vi "Measure.vi"(0 "eye scan single point":refnum<class "niHighSpeedSerial Eye Scan Single Point v1 Host.lvclass">, 5 "timeout (100 ms)":dbl=0.1, 11 "error in":errorcluster) -> (4 "eye scan single point out":refnum<class "niHighSpeedSerial Eye Scan Single Point v1 Host.lvclass">, 6 "bit error ratio":dbl, 8 "sample count":u64, 10 "error count":u64, 13 "timed out?":bool, 14 "done?":bool, 15 "error out":errorcluster)   [LabVIEW 2014, in "niHighSpeedSerial Eye Scan Single Point v1 Host.lvclass"]
doc: "Returns the Bit Error Rate, sample count, and error count on the point previously specified.\nThis VI returns under the following conditions, whichever comes first:\n1) The Eye Scan engine has completed measuring the point.\n2) The <b>timeout</b> is reached.\n\n<B>Input Parameters</B>\n\n<B>eye scan single point</B> takes in a reference to your session from the previous VI.\n\n<B>timeout (100 ms)</B> The amount of time (in seconds) before timing timing out.\nSpecifying '-1' prevents 'timed out' from ever returning true.\n\n<B>error in</B> describes error conditions that occur before this node runs. This input provides standard 'error in' functionality.\n\n<B>Output Parameters</B>\n\n<B>eye scan single point out</B> passes a reference to your session to the next VI.\n\n<B>bit error rate</B> is the calculated statistical bit error rate based on the number of error counts and sample counts received.\n\n<B>sample count</B> is the number of samples that have been measured on this point.\n\n<B>error count</B> is the number of errors that have been measured on this point.\n\n<B>timed out?</B> returns true if at least 'timeout' amount of time has passed.\n\n<B>done?</B> returns true if the Eye Scan algorithm has completed measuring all points.\n\n<B>error out</B> contains error information. This output provides standard 'error out' functionality."
uses:
  <instrlib>/niHighSpeedSerial/Eye Scan/v1/Host/Impl/Single Point/niHighSpeedSerial Eye Scan Single Point v1 Host.lvclass
  <instrlib>/niHighSpeedSerial/Eye Scan/v1/Host/Impl/Single Point/niHighSpeedSerial Eye Scan Single Point v1 Host.lvclass/niHighSpeedSerial Eye Scan Single Point v1 Host.ctl
  <vilib>/Utility/error.llb/Error Cluster From Error Code.vi
  <vilib>/ErrorRing/Error Ring.xnode
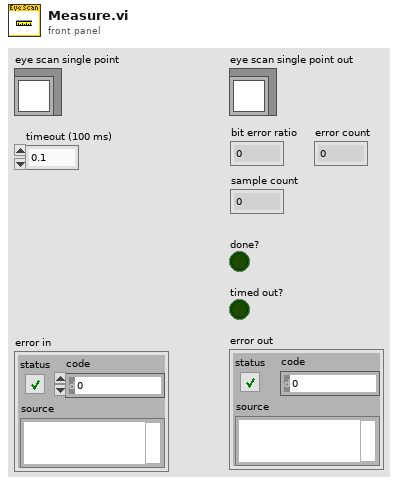
[diagram p1: front panel]
types:
  T1 = typedef "niHighSpeedSerial Eye Scan Single Point v1 Host.lvclass/Private Data.ctl" = cluster{"GTX2_CHANNEL register map":refnum<class "GTX2_CHANNEL Register Map.lvclass">, "instruction target":refnum<class "niInstr Instruction Target v1 Host.lvclass">, "channel measure state":T2, "in DFE mode?":bool, "prescale":u8, "receiver data width":T3, "active point":T4, "ut sign":T5, "positive counts":T6, "negative counts":T6}
  T2 = typedef "niHighSpeedSerial Eye Scan Single Point v1 Host.lvclass/Channel Measure State.ctl" = enum16{"Uninitialized", "Initialized", "Ready", "Request", "Wait", "Read", "Process", "Finished"}
  T3 = typedef "niHighSpeedSerial Eye Scan Common v1 Host.lvlib/Data Width.ctl" = enum16{"16 Bit", "20 Bit", "32 Bit", "40 Bit"}
  T4 = typedef "niHighSpeedSerial Eye Scan Common v1 Host.lvlib/Point Offsets.ctl" = cluster{"horizontal offset":i16, "vertical offset":i8}
  T5 = typedef "GTX2_CHANNEL v1 Host.lvlib/ESVertOffsetSign.ctl" = enum8{"Positive", "Negative"}
  T6 = typedef "niHighSpeedSerial Eye Scan Single Point v1 Host.lvclass/Counts.ctl" = cluster{"sample count":u64, "error count":u16}
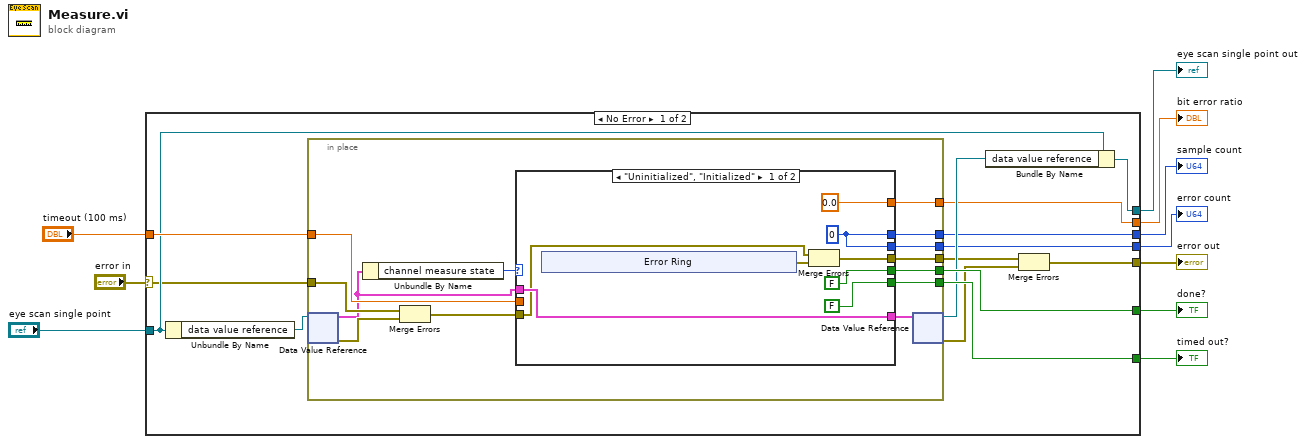
[diagram p0: block diagram]
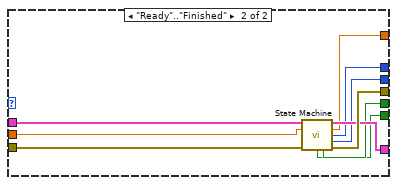
[diagram p2: hidden frame]
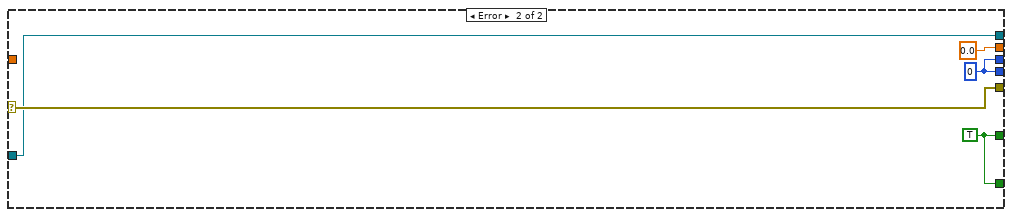
[diagram p3: hidden frame]
diagram:
  n1 = case shown="No Error" "error in" {
    selector: "error in" -> [w17 w64]
    tunnel: [w14 w64] -> w9
    tunnel: "timeout (100 ms)" -> [w24 _]
    tunnel: [w18 w63] -> w7
    tunnel: "eye scan single point" -> [w20 w63]
    tunnel: [w22 w62] -> w5
    tunnel: [w23 w62] -> w4
    tunnel: [w13 w61] -> w3
    tunnel: [w12 w61] -> w2
    tunnel: [w11 0.0 ("bit error ratio")] -> w1
    frame No Error {
      n2 = Unbundle By Name(w20) -> ("data value reference"=w21:refnum<data-value>)
      n3 = in-place {
        in-place-border: [w34] -> w15
        in-place-border: w24 -> [w33]
        in-place-border: [w30] -> w23
        in-place-border: [w31] -> w22
        in-place-border: w17 -> [w37]
        in-place-border: [w27] -> w13
        in-place-border: [w26] -> w12
        in-place-border: [w25] -> w11
        n4 = in-place-dvr #1(w21) -> (w29:T1, w36:errorcluster)
        n5 = Unbundle By Name(w29) -> ("channel measure state"=w28:T2)
        n6 = Merge Errors(w37, w36) -> (w35:errorcluster)
        n7 = case shown="\"Uninitialized\", \"Initialized\"" w28 {
          tunnel: w35 -> [w42 w59]
          tunnel: [w41 w58] -> w34
          tunnel: w33 -> [_ w57]
          tunnel: [w45 w56] -> w32
          tunnel: [FALSE ("done") w54] -> w31
          tunnel: [FALSE ("Timed out?") w53] -> w30
          tunnel: w29 -> [w45 w55]
          tunnel: [w40 w52] -> w27
          tunnel: [w40 w51] -> w26
          tunnel: [0.0 ("bit error ratio") w50] -> w25
          frame "Uninitialized", "Initialized" {
            w40 = u64 0 ("sample count")
            n8 = xnode "Error Ring"() -> ("error out"=w38:errorcluster)
            n9 = Merge Errors(w42, w38) -> (w41:errorcluster)
          }
          frame "Ready".."Finished" {
            n10 = call <instrlib>:"State Machine.vi"("private data"=w55, "timeout (100 ms)"=w57, "error in"=w59) -> ("private data out"=w56:T1, "bit error rate"=w50:dbl, "sample count"=w51:u64, "error count"=w52:u64, "timed out?"=w53:bool, "done?"=w54:bool, "error out"=w58:errorcluster)  [unwired: 6 in]
          }
        }
        n11 = in-place-dvr #1(w32) -> (w19:refnum<data-value>, w16:errorcluster)
      }
      n12 = Bundle By Name(cluster=w20, "data value reference"=w19) -> (w18:refnum<class "niHighSpeedSerial Eye Scan Single Point v1 Host.lvclass">)
      n13 = Merge Errors(w15, w16) -> (w14:errorcluster)
    }
    frame Error {
      w61 = u64 0 ("error count")
      w62 = TRUE ("done")
    }
  }
  "eye scan single point out" <- w7
  "error out" <- w9
  "done?" <- w5
  "timed out?" <- w4
  "bit error ratio" <- w1
  "sample count" <- w2
  "error count" <- w3
